vi "onSuiteSlippage.vi"(7 "TraceabilityMatrix in":refnum<class "TraceabilityMatrix.lvclass">, 11 "Leaf.TestSuite":refnum<class "Leaf.TestSuite.lvclass">) -> (0 "error out":errorcluster, 3 "Leaf.TestSuite":refnum<class "Leaf.TestSuite.lvclass">)   [LabVIEW 2021, in "Bananas.lvlib" / "TraceabilityMatrix.lvclass"]
uses:
  TraceabilityMatrix.lvclass
  Leaf.TestSuite/Leaf.TestSuite.lvclass
  TraceabilityMatrix.lvclass/TraceabilityMatrix.ctl
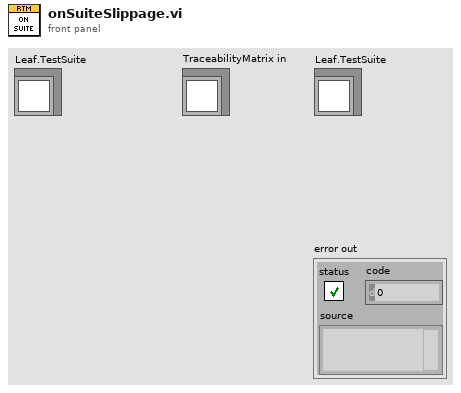
[diagram p1: front panel]
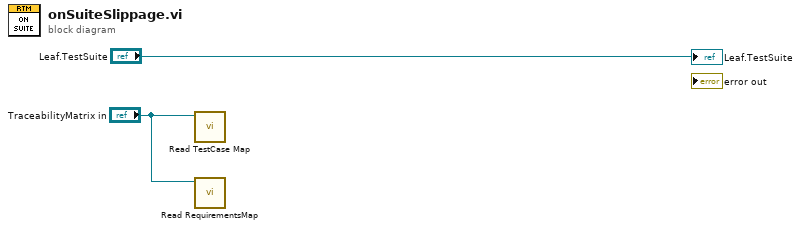
[diagram p0: block diagram]
diagram:
  n1 = call "Read TestCase Map.vi"("TraceabilityMatrix in"="TraceabilityMatrix in") -> ()  [unwired: 9 in, 2 out]
  n2 = call "Read RequirementsMap.vi"("TraceabilityMatrix in"="TraceabilityMatrix in") -> ()  [unwired: 9 in, 2 out]
  "Leaf.TestSuite" <- "Leaf.TestSuite"
